vi "Command_SetRobotPose.vi"(7 "Parameters":dbl[](array[numeric]), 11 "Startup":bool) -> (4 "Completed":bool, 15 "Reinit":bool)   [LabVIEW 2020]
uses:
  Auto Utilities/Command_Execution_State.ctl
  Globals/Drive_Globals.vi
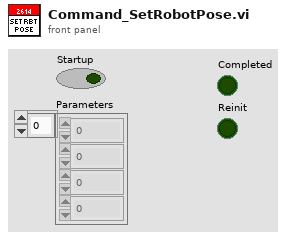
[diagram p1: front panel]
types:
  T1 = typedef "Command_Execution_State.ctl" = enum16{"Initialize", "Execute", "Finish"}
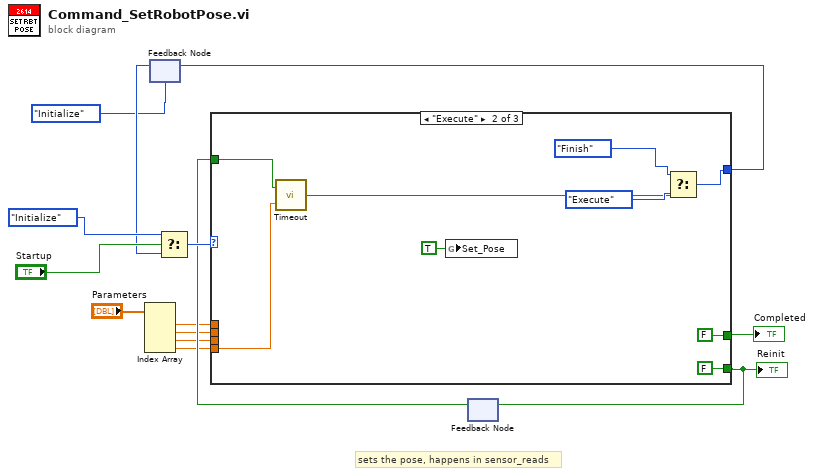
[diagram p0: block diagram]
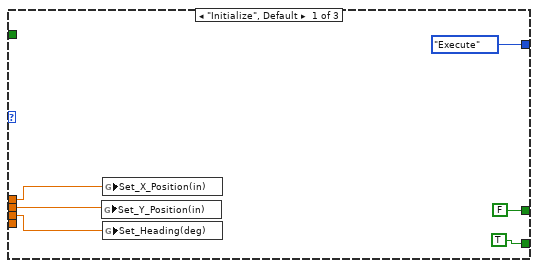
[diagram p2: hidden frame]
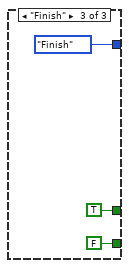
[diagram p3: hidden frame]
diagram:
  # "sets the pose, happens in sensor_reads"
  n1 = Index Array(array="Parameters") -> (element #1=w4:dbl, element #2=w3:dbl, element #3=w2:dbl, element #4=w1:dbl)  [unwired: 4 in]
  n2 = feedback #1(Command_Execution_State."Initialize") -> (w10:T1)
  n3 = Select(t=Command_Execution_State."Initialize", s="Startup", f=w10) -> (s? t:f=w12:T1)
  n4 = feedback #2() -> (w6:bool)  [unwired: 1 in]
  n5 = case shown="\"Execute\"" w12 {
    tunnel: [Command_Execution_State."Execute" w24 Command_Execution_State."Finish"] -> w11
    tunnel: [FALSE ("Reinit") FALSE ("Reinit") TRUE ("Reinit")] -> w8
    tunnel: [TRUE ("Reinit") FALSE ("Reinit") FALSE ("Reinit")] -> w7
    tunnel: w6 -> [_ w21 _]
    tunnel: w4 -> [w17 _ _]
    tunnel: w3 -> [w16 _ _]
    tunnel: w2 -> [w15 _ _]
    tunnel: w1 -> [_ w27 _]
    frame "Initialize", Default {
      n6 = global write "Drive_Globals.vi" "Set_Y_Position(in)"(w16) -> ()
      n7 = global write "Drive_Globals.vi" "Set_X_Position(in)"(w17) -> ()
      n8 = global write "Drive_Globals.vi" "Set_Heading(deg)"(w15) -> ()
    }
    frame "Execute" {
      n9 = call "Timeout.vi"("Timeout"=w27, "Initialize"=w21) -> ("Timed Out?"=w23:bool)
      n10 = global write "Drive_Globals.vi" "Set_Pose"(TRUE ("Set_Pose")) -> ()
      n11 = Select(t=Command_Execution_State."Finish", s=w23, f=Command_Execution_State."Execute") -> (s? t:f=w24:T1)
    }
    frame "Finish" {
    }
  }
  "Reinit" <- w7
  "Completed" <- w8
  n12 = feedback-in #1(w11) -> ()
  n13 = feedback-in #2(w7) -> ()
